vi "load modules.vi"() -> ()   [LabVIEW 2017]
doc: "SciScan 1.2 160622"
uses:
  GFG/GFGstringGet.vi
  GFG/GFG library.lvlib
panel:
  out "Array":T1(array[cluster])
  out "error out":errorcluster
  in  "error in (no error)":errorcluster
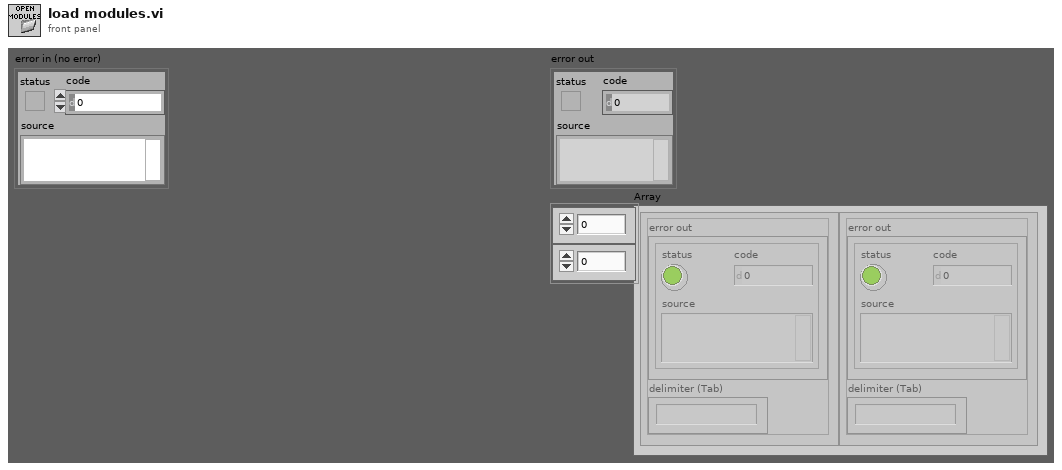
[diagram p1: front panel]
types:
  T1 = cluster{"error out":errorcluster, "delimiter (Tab)":string}[][]
  T2 = enum32{"Invalid", "Standard", "Closed", "Hidden", "Minimized", "Maximized"}
  T3 = cluster{"error out":errorcluster, "delimiter (Tab)":string}
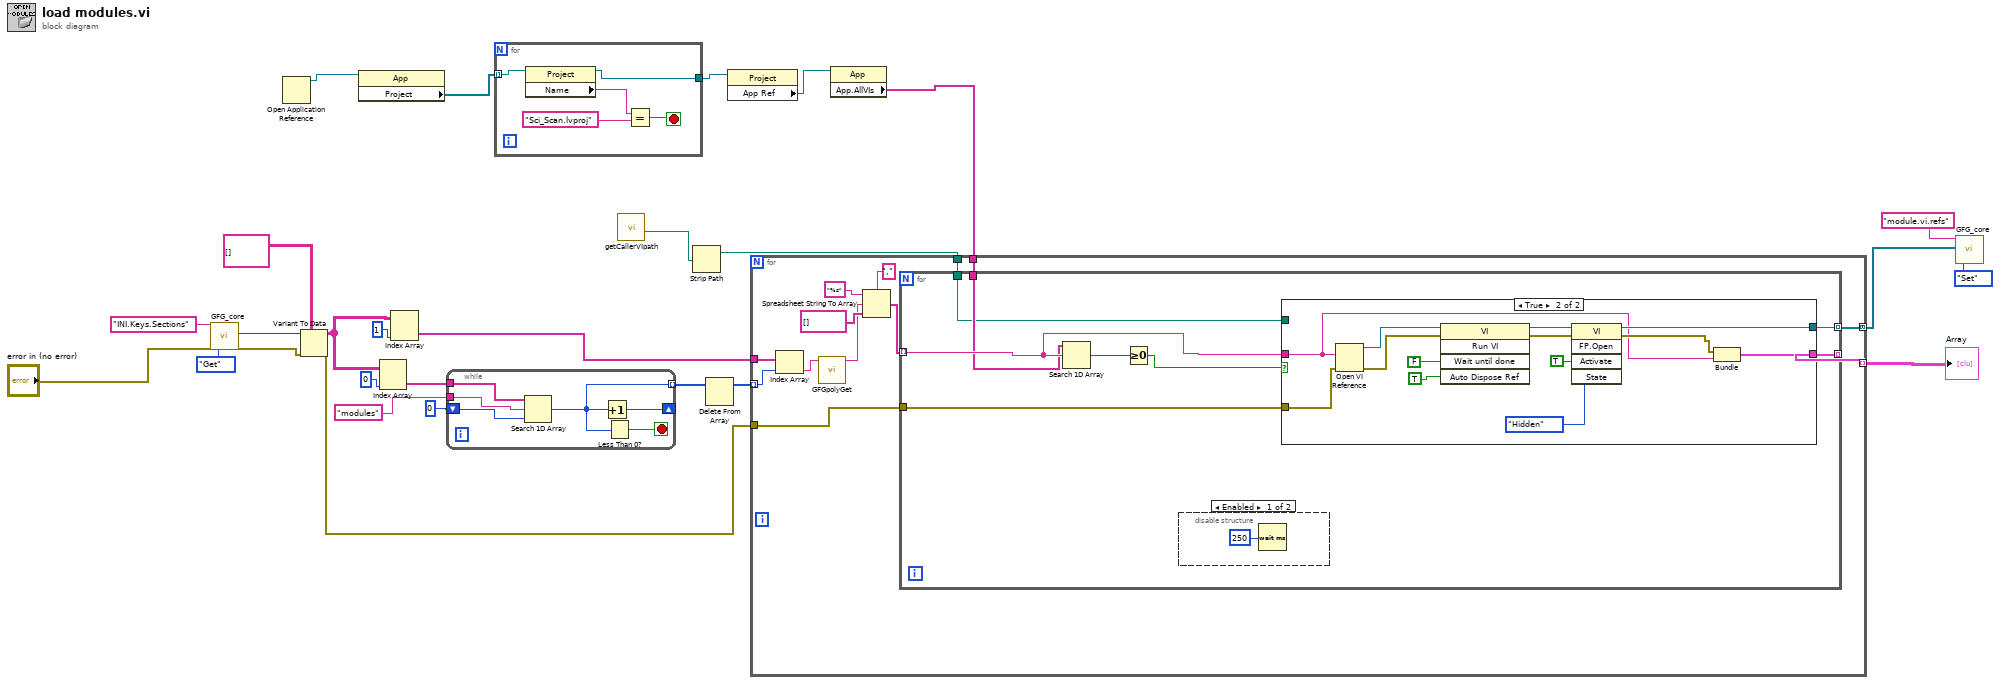
[diagram p0: block diagram]
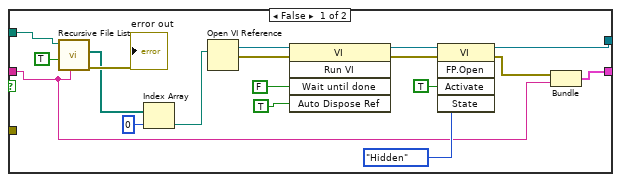
[diagram p3: hidden frame]
diagram:
  n1 = call "GFG_core.vi"("Variable Name in"="INI.Keys.Sections", "error in (no error)"="error in (no error)", "Action"=enum16{"Init", "Set", "Get"}."Get") -> ("Variant Out"=w25:variant, "error out"=w13:errorcluster)  [unwired: 10 in, 5 out]
  n2 = Open Application Reference() -> (3:w2:refnum<vi>)  [unwired: 4 in, 1 out]
  n3 = Variant To Data(error in=w13, type=string[][] [], Variant=w25) -> (data=w21:string[][], error out=w12:errorcluster)
  n4 = property class="App"(reference=w2) -> ("Project"=w3:refnum<vi>[])  [unwired: 1 in, 2 out]
  n5 = Index Array(array=w21, index (col)=0 ("index (row)")) -> (element=w23:string[])  [unwired: 1 in]
  n6 = Index Array(array=w21, index (col)=1 ("index (row)")) -> (element=w20:string[])  [unwired: 1 in]
  n7 = while {
    tunnel: w23 -> [w33]
    shift-right: [w30] -> _
    shift-left: 0 ("index of element") -> [w32]
    tunnel: [w29] -> w16 mode=indexing
    tunnel: "modules" ("element") -> [w28]
    stop <- w31 stop-if-true
    n8 = Search 1D Array(1D array=w33, element=w28, start index (0)=w32) -> (index of element=w29:i32)
    n9 = Increment(x=w29) -> (x+1=w30:i32)
    n10 = Less Than 0?(x=w29) -> (x < 0?=w31:bool)
  }
  n11 = for {
    tunnel: w3 -> [w38] mode=indexing
    tunnel: [w35] -> w4
    stop <- w34 stop-if-true
    n12 = property class="Project"(reference=w38) -> (reference out=w35:refnum<vi>, "Name"=w36:string)  [unwired: 1 in, 1 out]
    n13 = Equal?(x=w36, y="Sci_Scan.lvproj" ("Name")) -> (x = y?=w34:bool)
  }
  n14 = call "getCallerVIpath.vi"() -> ("calling VI's  parent path"=w7:path)  [unwired: 10 in, 1 out]
  n15 = Strip Path(path=w7) -> (stripped path=w6:path)  [unwired: 1 out]
  n16 = Delete From Array(array=w16) -> (array with subset deleted=w15:i32[])  [unwired: 2 in, 1 out]
  n17 = property class="Project"(reference=w4) -> ("App Ref"=w5:refnum<vi>)  [unwired: 1 in, 2 out]
  n18 = property class="App"(reference=w5) -> ("App.AllVIs"=w1:string[])  [unwired: 1 in, 2 out]
  n19 = for {
    tunnel: w20 -> [w51]
    tunnel: w15 -> [w50] mode=indexing
    tunnel: w12 -> [w49]
    tunnel: [w42] -> w10 mode=concatenating
    tunnel: w6 -> [w41]
    tunnel: [w40] -> w8 mode=indexing
    tunnel: w1 -> [w39]
    n20 = Index Array(array=w51, index=w50) -> (element=w44:string)
    n21 = call-poly "GFGpolyGet.vi"("Variable Name in"=w44) -> ("String"=w43:string)  [unwired: 9 in, 1 out]
    n22 = Spreadsheet String To Array(delimiter (Tab)=",", format string="%s" ("Variable Name in"), spreadsheet string=w43, array type (2D Dbl)=string[] [] ("Array")) -> (array=w45:string[])
    n23 = for {
      tunnel: w49 -> [w54]
      tunnel: w45 -> [w57] mode=indexing
      tunnel: [w59] -> w42 mode=indexing
      tunnel: w41 -> [w53]
      tunnel: [w58] -> w40 mode=indexing
      tunnel: w39 -> [w56]
      n24 = Search 1D Array(1D array=w56, element=w57) -> (index of element=w52:i32)  [unwired: 1 in]
      n25 = Greater Or Equal To 0?(x=w52) -> (x >= 0?=w55:bool)
      n26 = disable-structure shown="Enabled" {
        frame Enabled {
          n27 = Wait (ms)(milliseconds to wait=u32 250) -> ()  [unwired: 1 out]
        }
        frame Disabled {
        }
      }
      n28 = case shown="True" w55 {
        tunnel: w54 -> [_ w88]
        tunnel: [w62 w87] -> w59
        tunnel: [w61 w86] -> w58
        tunnel: w57 -> [w63 w80]
        tunnel: w53 -> [w74 _]
        frame False {
          n29 = call <vilib>:"Recursive File List.vi"("pattern"=w63, "Continue Recursing on Error? (F)"=TRUE, "Folder Path"=w74) -> ("error out"=→"error out":errorcluster, "All Files in Dir"=w76:path[])  [unwired: 4 in, 3 out]
          n30 = Index Array(array=w76, index=0) -> (element=w64:path)
          n31 = Open VI Reference(vi path=w64) -> (vi reference=w68:refnum<vi>, error out=w73:errorcluster)  [unwired: 5 in]
          n32 = invoke class="VI" method="Run VI"(reference=w68, error in=w73, "Wait until done"=FALSE, "Auto Dispose Ref"=TRUE ("Auto Dispose Reference")) -> (reference out=w66:refnum<vi>, error out=w71:errorcluster)  [unwired: 1 in, 3 out]
          n33 = invoke class="VI" method="FP.Open"(reference=w66, error in=w71, "Activate"=TRUE ("Activate?"), "State"=T2."Hidden") -> (reference out=w62:refnum<vi>, error out=w72:errorcluster)  [unwired: 1 in, 3 out]
          n34 = Bundle("error out"=w72, "delimiter (Tab)"=w63) -> (w61:T3)  [unwired: 1 in]
        }
        frame True {
          n35 = Open VI Reference(vi path=w80, error in (no error)=w88) -> (vi reference=w79:refnum<vi>, error out=w81:errorcluster)  [unwired: 4 in]
          n36 = invoke class="VI" method="Run VI"(reference=w79, error in=w81, "Wait until done"=FALSE, "Auto Dispose Ref"=TRUE ("Auto Dispose Reference")) -> (reference out=w90:refnum<vi>, error out=w83:errorcluster)  [unwired: 1 in, 3 out]
          n37 = invoke class="VI" method="FP.Open"(reference=w90, error in=w83, "Activate"=TRUE ("Activate?"), "State"=T2."Hidden") -> (reference out=w87:refnum<vi>, error out=w82:errorcluster)  [unwired: 1 in, 3 out]
          n38 = Bundle("error out"=w82, "delimiter (Tab)"=w80) -> (w86:T3)  [unwired: 1 in]
        }
      }
    }
  }
  "Array" <- w8
  n39 = call "GFG_core.vi"("Variable Name in"="module.vi.refs", "Variant in"=w10, "Action"=enum16{"Init", "Set", "Get"}."Set") -> ()  [unwired: 10 in, 7 out]
